vi "Report.vi"() -> ()   [LabVIEW 2020, in "Database Lib.lvlib"]
uses:
  Database Lib.lvlib
  <vilib>/Utility/miscctls.llb/LVRowAndColumnTypeDef.ctl
  <vilib>/Utility/NIReport.llb/Report Type.ctl
  <vilib>/addons/_office/_exclsub.llb/font.ctl
  <vilib>/addons/_office/excel.llb/Excel Easy Table (str).vi
  <vilib>/Utility/NIReport.llb/NI_report.lvclass
  <vilib>/Utility/NIReport.llb/NI_ReportGenerationCore.lvlib
  <vilib>/addons/_office/NI_ReportGenerationToolkit.lvlib
  <vilib>/Utility/NIReport.llb/Excel/NI_Excel.lvclass
panel:
  out "Grading Data":string[][](array[string])
  in  "Menu":enum32{"Log Catalog", "Log", "Grading"}(radio)
  out "Tab Control":enum32{"Log Catalog", "Log", "Grading"}(tab)
  in  "Search Log Catalog Table":bool
  out "Log Catalog Table":string[][](table)
  out "Log Table":string[][](table)
  in  "Save Log Table":bool
  in  "Search Log Table":bool
  in  "Catalog ID Log Table 2":u16 caption="Catalog ID" max=9999 step=1 format="%04.0f"
  in  "To Catalog ID Log Table":bool
  in  "Until Hour Log Table":u8 caption="Hour" max=23 step=1 format="%02.0f"
  in  "Until Minute Log Table":u8 caption="Minute" max=59 step=1 format="%02.0f"
  in  "Until Second Log Table":u8 caption="Second" max=59 step=1 format="%02.0f"
  in  "Until Time Log Table":bool
  in  "Since Time Log Table":bool
  in  "Until Date Log Table":bool
  in  "Until Year Log Table":u16 caption="Year" format="%04.0f"
  in  "Until Month Log Table":u8 caption="Month" max=12 step=1 format="%02.0f"
  in  "Until Day Log Table":u8 caption="Day" max=31 step=1 format="%02.0f"
  in  "Catalog ID Log Table 1":u16 caption="Catalog ID" max=9999 step=1 format="%04.0f"
  in  "Since Year Log Table":u16 caption="Year" format="%04.0f"
  in  "Since Month Log Table":u8 caption="Month" max=12 step=1 format="%02.0f"
  in  "Since Day Log Table":u8 caption="Day" max=31 step=1 format="%02.0f"
  in  "Since Hour Log Table":u8 caption="Hour" max=23 step=1 format="%02.0f"
  in  "Since Minute Log Table":u8 caption="Minute" max=59 step=1 format="%02.0f"
  in  "Since Second Log Table":u8 caption="Second" max=59 step=1 format="%02.0f"
  in  "Since Date Log Table":bool
  in  "From Catalog ID Log Table":bool
  out "Grading Table":string[][](table)
  in  "Search Grading Table":bool
  in  "Save Grading Table":bool
  in  "From Test Number":bool
  in  "Since Date Grading Table":bool
  in  "Since Second Grading Table":u8 caption="Second" max=59 step=1 format="%02.0f"
  in  "Since Minute Grading Table":u8 caption="Minute" max=59 step=1 format="%02.0f"
  in  "Since Hour Grading Table":u8 caption="Hour" max=23 step=1 format="%02.0f"
  in  "Since Day Grading Table":u8 caption="Day" max=31 step=1 format="%02.0f"
  in  "Since Month Grading Table":u8 caption="Month" max=12 step=1 format="%02.0f"
  in  "Since Year Grading Table":u16 caption="Year" format="%04.0f"
  in  "Test Number 1":u64 caption="Test Number" max=9999 step=1 format="%010.0f"
  in  "Until Day Grading Table":u8 caption="Day" max=31 step=1 format="%02.0f"
  in  "Until Month Grading Table":u8 caption="Month" max=12 step=1 format="%02.0f"
  in  "Until Year Grading Table":u16 caption="Year" format="%04.0f"
  in  "Until Date Grading Table":bool
  in  "Since Time Grading Table":bool
  in  "Until Time Grading Table":bool
  in  "Until Second Grading Table":u8 caption="Second" max=59 step=1 format="%02.0f"
  in  "Until Minute Grading Table":u8 caption="Minute" max=59 step=1 format="%02.0f"
  in  "Until Hour Grading Table":u8 caption="Hour" max=23 step=1 format="%02.0f"
  in  "To Test Number":bool
  in  "Test Number 2":u64 caption="Catalog ID" max=9999 step=1 format="%010.0f"
  in  "Graphs Grading Table":bool
  in  "Close":bool
  # "/"
  # "/"
  # ":"
  # ":"
  # "/"
  # "/"
  # ":"
  # ":"
  # "/"
  # "/"
  # ":"
  # ":"
  # "/"
  # "/"
  # ":"
  # ":"
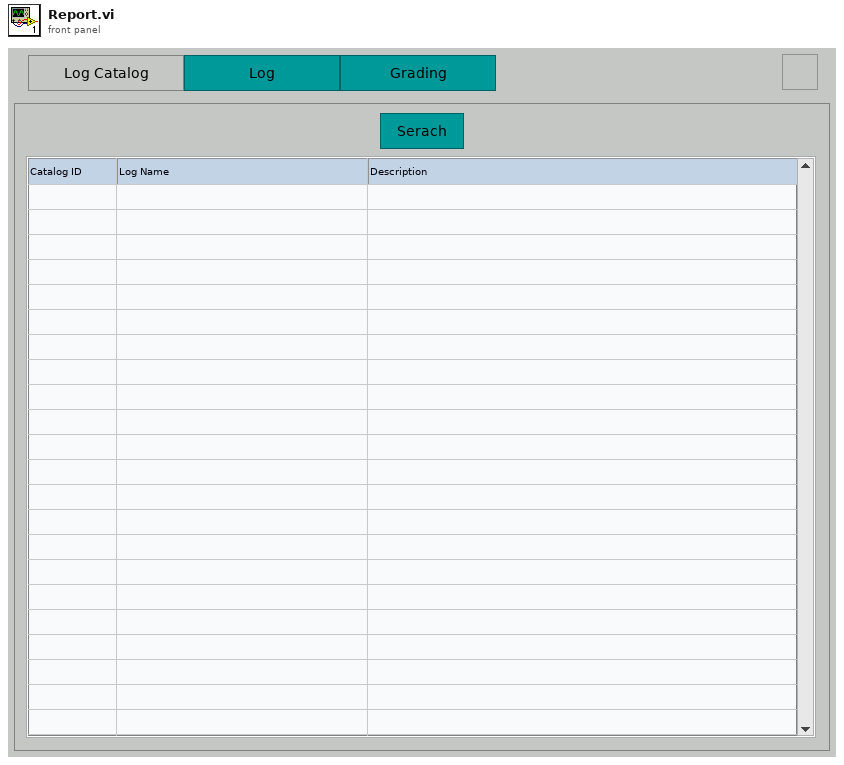
[diagram p1: front panel]
types:
  T1 = typedef "LVRowAndColumnTypeDef.ctl" = cluster{"Row":i32, "Column":i32}
  T2 = typedef "NI_ReportGenerationToolkit.lvlib/font.ctl" = cluster{"font name":string, "font size":dbl, "bold":u16, "italic":u16, "underline":u16, "strike through":u16, "font color":u32}
  T3 = enum16{"maximized", "minimized", "normal", "no change"}
  T4 = typedef "NI_ReportGenerationCore.lvlib/Report Type.ctl" = enum16{"HTML", "Word", "Excel"}
  T5 = cluster{"Since Year Grading Table":u16, "Since Month Grading Table":u8, "Since Day Grading Table":u8, "Until Year Grading Table":u16, "Until Month Grading Table":u8, "Until Day Grading Table":u8, "Since Date Grading Table":bool, "Until Date Grading Table":bool}
  T6 = cluster{"Since Hour Grading Table":u8, "Since Minute Grading Table":u8, "Since Second Grading Table":u8, "Until Hour Grading Table":u8, "Until Minute Grading Table":u8, "Until Second Grading Table":u8, "Since Time Grading Table":bool, "Until Time Grading Table":bool}
  T7 = cluster{"Test Number 1":u64, "Test Number 2":u64, "From Test Number":bool, "To Test Number":bool}
  T8 = cluster{"Since Year Log Table":u16, "Since Month Log Table":u8, "Since Day Log Table":u8, "Until Year Log Table":u16, "Until Month Log Table":u8, "Until Day Log Table":u8, "Since Date Log Table":bool, "Until Date Log Table":bool}
  T9 = cluster{"Since Hour Log Table":u8, "Since Minute Log Table":u8, "Since Second Log Table":u8, "Until Hour Log Table":u8, "Until Minute Log Table":u8, "Until Second Log Table":u8, "Since Time Log Table":bool, "Until Time Log Table":bool}
  T10 = cluster{"Catalog ID Log Table 1":u16, "Catalog ID Log Table 2":u16, "From Catalog ID Log Table":bool, "To Catalog ID Log Table":bool}
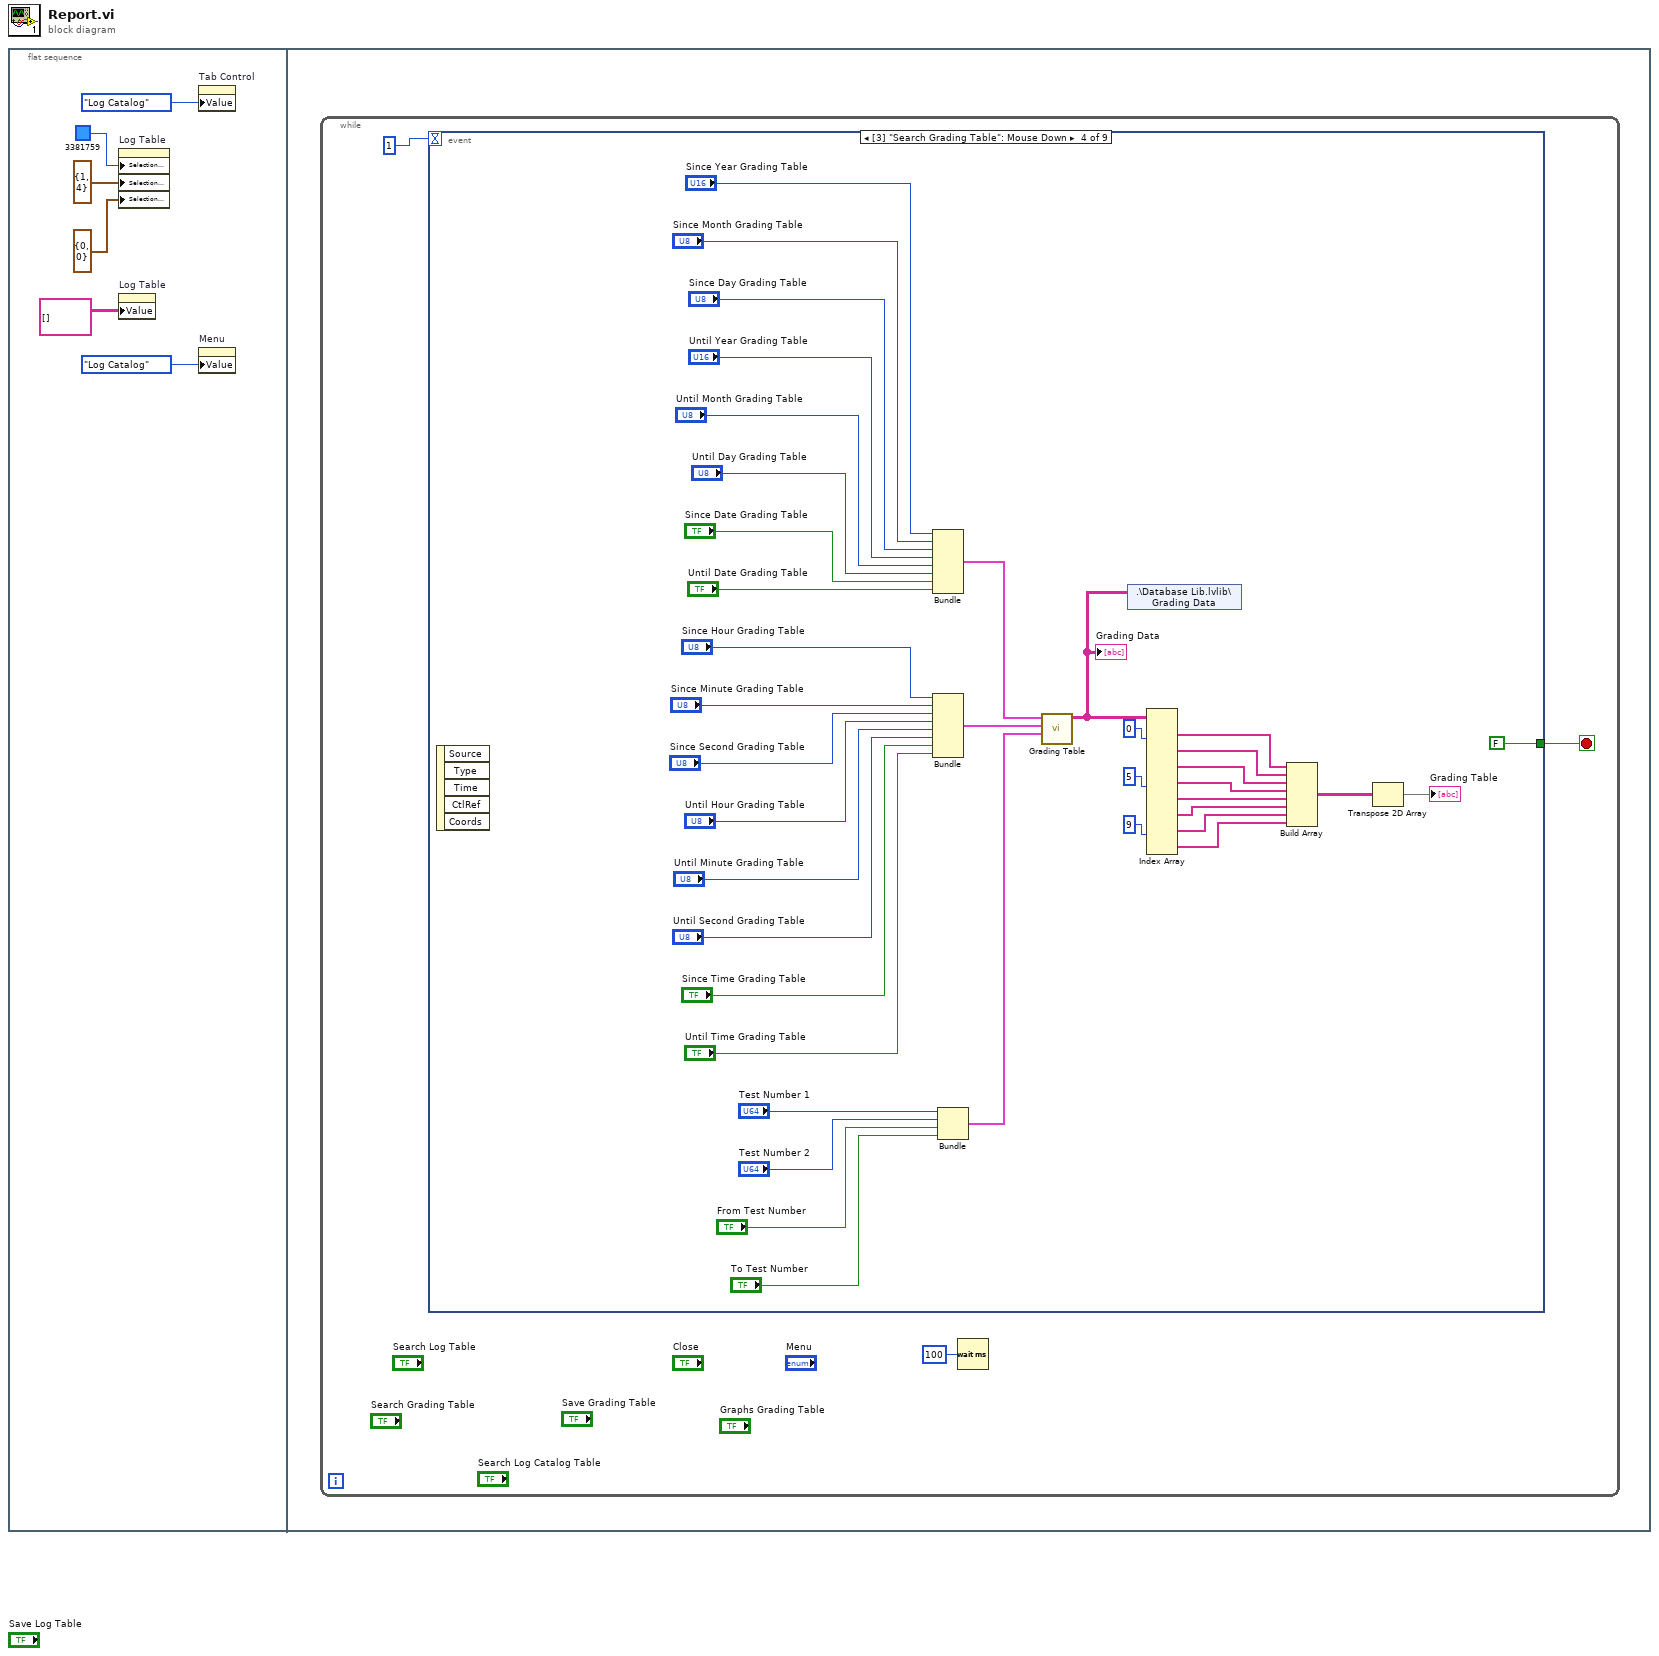
[diagram p0: block diagram]
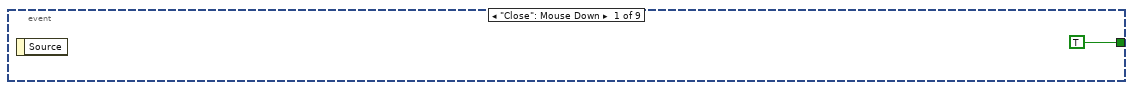
[diagram p2: hidden frame]
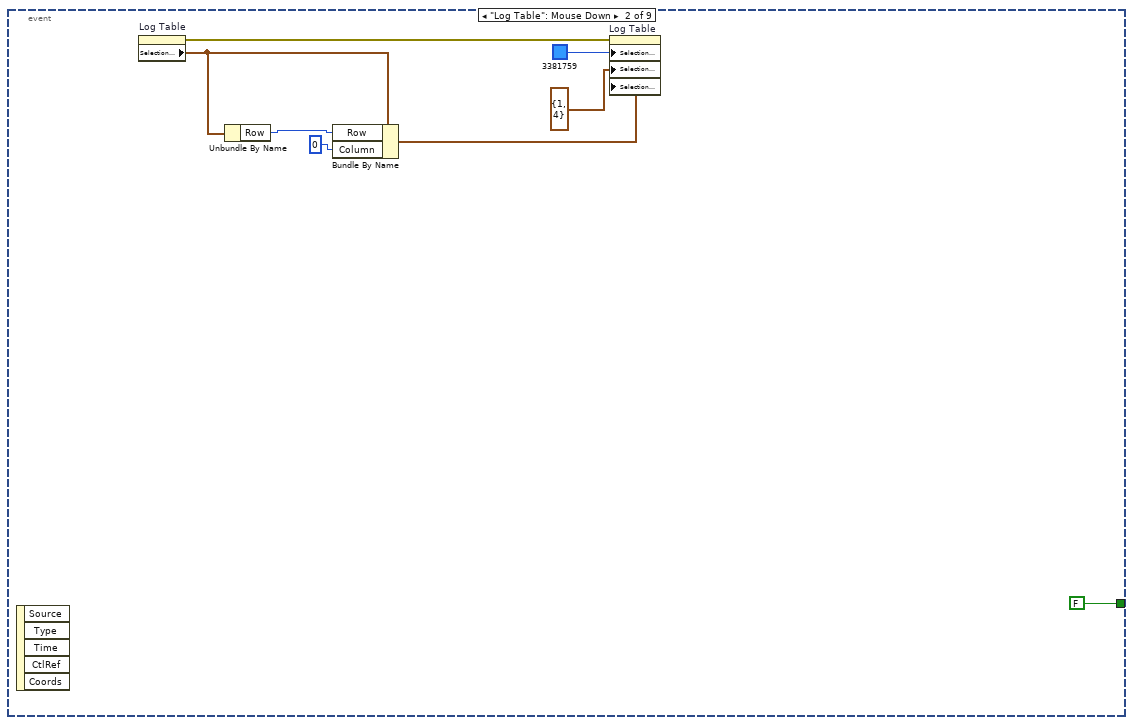
[diagram p3: hidden frame]
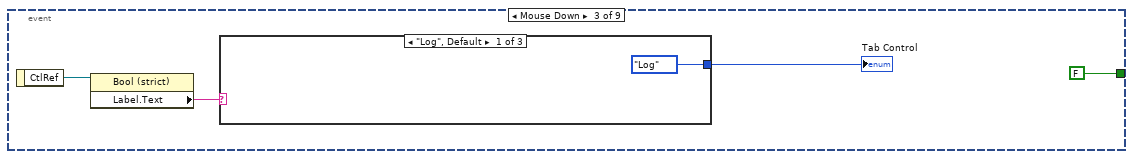
[diagram p4: hidden frame]
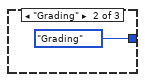
[diagram p5: hidden frame]
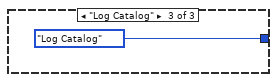
[diagram p6: hidden frame]
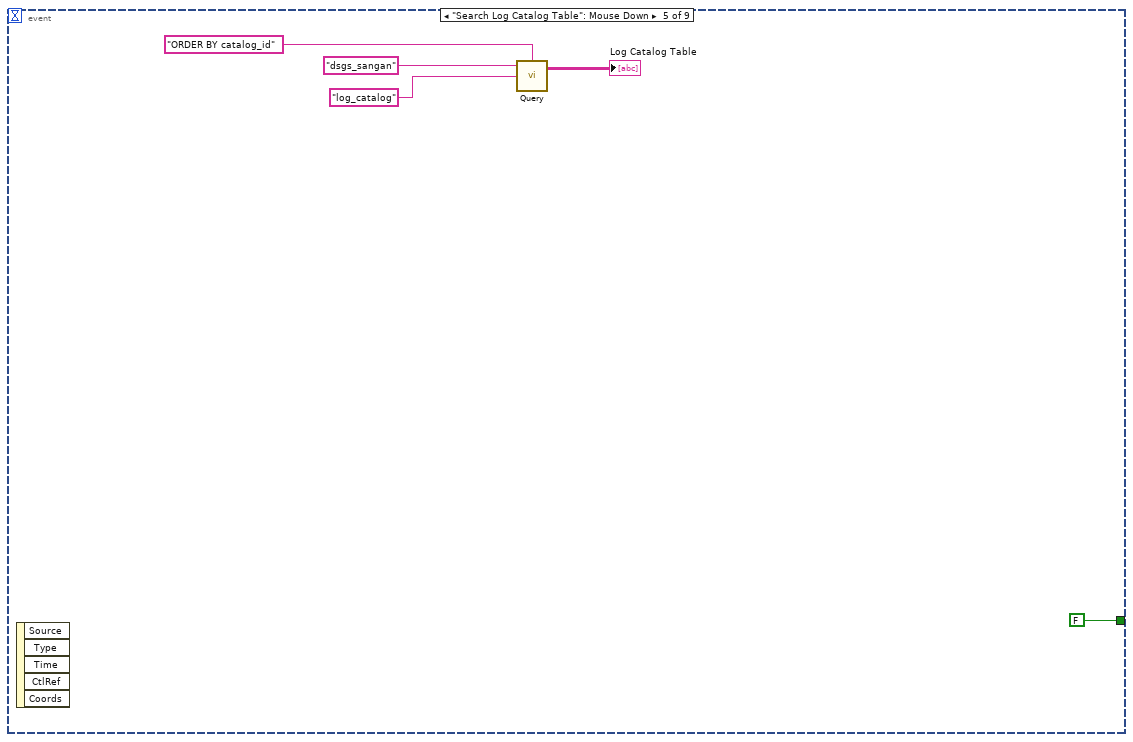
[diagram p7: hidden frame]
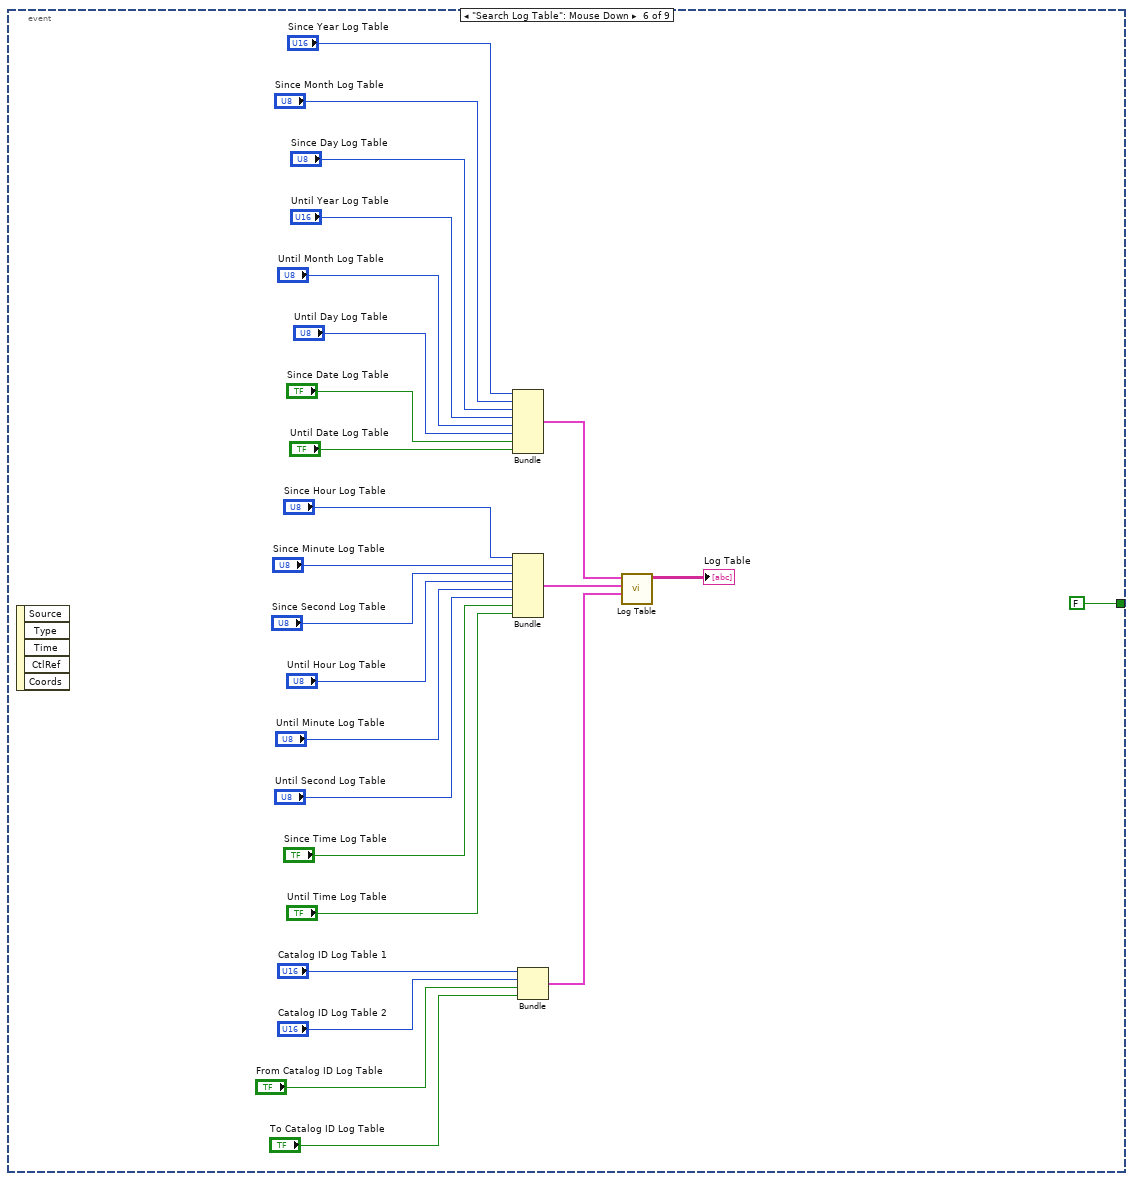
[diagram p8: hidden frame]
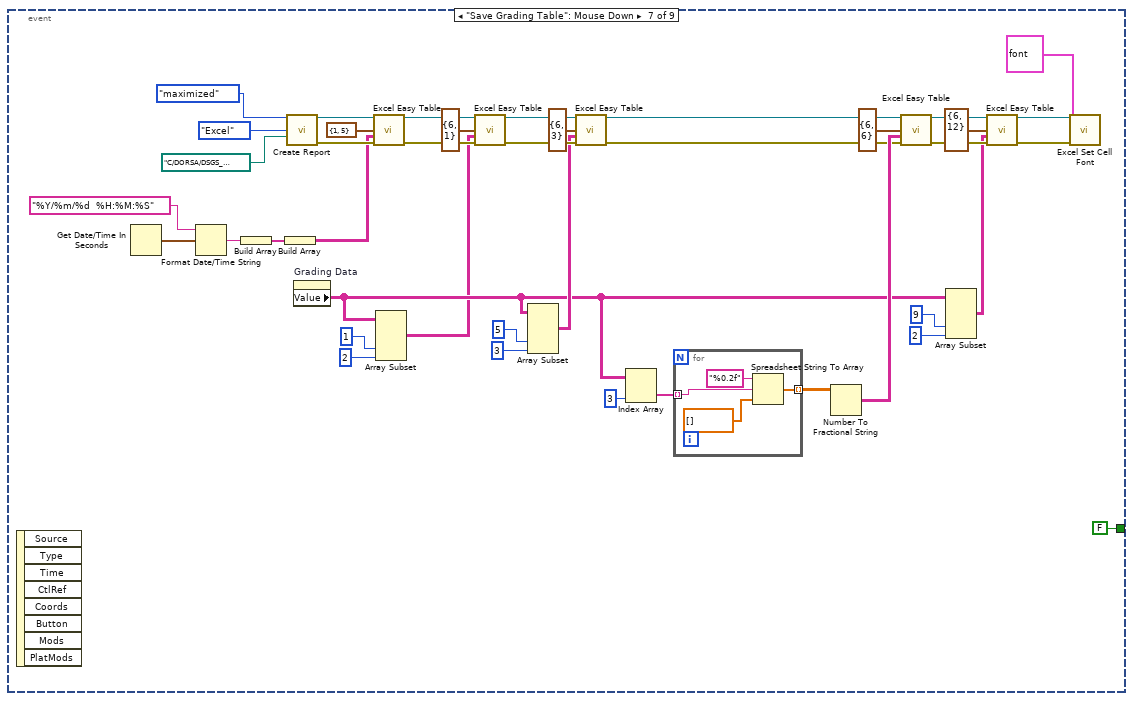
[diagram p9: hidden frame]
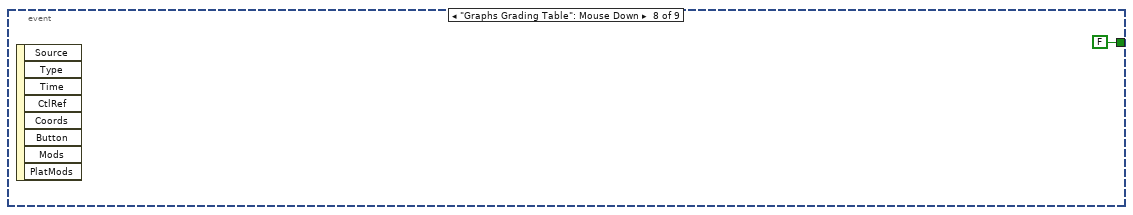
[diagram p10: hidden frame]
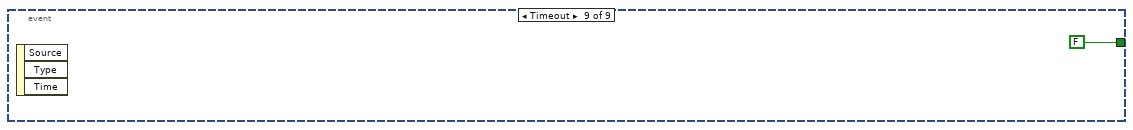
[diagram p11: hidden frame]
diagram:
  n1 = flat-sequence {
    frame #0 {
      n2 = property on="Log Table" class="Tbl (strict)"("Selection Color"=u32 3381759, "Selection Size"=T1 {"Row"=1, "Column"=4}, "Selection Start"=T1 {"Row"=0, "Column"=0}) -> ()  [unwired: 2 in, 2 out]
      n3 = property on="Log Table" class="Tbl (strict)"("Value"=string[][] []) -> ()  [unwired: 2 in, 2 out]
      n4 = property on="Tab Control" class="TabCtl (strict)"("Value"=enum32{"Log Catalog", "Log", "Grading"}."Log Catalog" ("Tab Control")) -> ()  [unwired: 2 in, 2 out]
      n5 = property on="Menu" class="RadioBtnsControl (strict)"("Value"=enum32{"Log Catalog", "Log", "Grading"}."Log Catalog" ("Menu")) -> ()  [unwired: 2 in, 2 out]
    }
    frame #1 {
      n6 = while {
        stop <- w9 stop-if-true
        n7 = event shown="[3] \"Search Grading Table\": Mouse Down" {
          selector: _ -> [_ _ _ _ _ _ _ _ _]
          dyn-events: _ -> [_ _ _ _ _ _ _ _ _]
          timeout: 1 -> [_ _ _ _ _ _ _ _ _]
          tunnel: [TRUE FALSE FALSE FALSE FALSE FALSE FALSE FALSE FALSE] -> w9
          event "Close": Mouse Down {
            n8 = event-data() -> ()  [unwired: 1 in, 1 out]
          }
          event "Log Table": Mouse Down {
            n9 = event-data() -> ()  [unwired: 1 in, 5 out]
            n10 = property on="Log Table" class="Tbl (strict)"() -> (error out=w16:errorcluster, "Selection Start"=w14:T1)  [unwired: 2 in, 1 out]
            n11 = Unbundle By Name(w14) -> ("Row"=w15:i32)
            n12 = Bundle By Name(cluster=w14, "Row"=w15, "Column"=0) -> (w17:T1)
            n13 = property on="Log Table" class="Tbl (strict)"(error in=w16, "Selection Color"=u32 3381759, "Selection Size"=T1 {"Row"=1, "Column"=4}, "Selection Start"=w17) -> ()  [unwired: 1 in, 2 out]
          }
          event "Menu.Log Catalog", "Menu.Log", "Menu.Grading": Mouse Down {
            n14 = event-data() -> ("CtlRef"=w21:refnum<vi>)  [unwired: 1 in]
            n15 = property class="Bool (strict)"(reference=w21) -> ("Label.Text"=w20:string)  [unwired: 1 in, 2 out]
            n16 = case shown="\"Log\", Default" w20 {
              tunnel: [enum32{"Log Catalog", "Log", "Grading"}."Log" ("Tab Control") enum32{"Log Catalog", "Log", "Grading"}."Grading" ("Tab Control") enum32{"Log Catalog", "Log", "Grading"}."Log Catalog" ("Tab Control")] -> w19
              frame "Log", Default {
              }
              frame "Grading" {
              }
              frame "Log Catalog" {
              }
            }
            "Tab Control" <- w19
          }
          event "Search Grading Table": Mouse Down {
            n17 = event-data() -> ()  [unwired: 1 in, 5 out]
            n18 = Bundle("Since Year Grading Table"="Since Year Grading Table", "Since Month Grading Table"="Since Month Grading Table", "Since Day Grading Table"="Since Day Grading Table", "Until Year Grading Table"="Until Year Grading Table", "Until Month Grading Table"="Until Month Grading Table", "Until Day Grading Table"="Until Day Grading Table", "Since Date Grading Table"="Since Date Grading Table", "Until Date Grading Table"="Until Date Grading Table") -> (w61:T5)  [unwired: 1 in]
            n19 = Bundle("Since Hour Grading Table"="Since Hour Grading Table", "Since Minute Grading Table"="Since Minute Grading Table", "Since Second Grading Table"="Since Second Grading Table", "Until Hour Grading Table"="Until Hour Grading Table", "Until Minute Grading Table"="Until Minute Grading Table", "Until Second Grading Table"="Until Second Grading Table", "Since Time Grading Table"="Since Time Grading Table", "Until Time Grading Table"="Until Time Grading Table") -> (w62:T6)  [unwired: 1 in]
            n20 = Bundle("Test Number 1"="Test Number 1", "Test Number 2"="Test Number 2", "From Test Number"="From Test Number", "To Test Number"="To Test Number") -> (w63:T7)  [unwired: 1 in]
            n21 = call "Grading Table.vi"("Test number"=w63, "Time"=w62, "Date"=w61) -> ("Grading Table"=w26:string[][])  [unwired: 7 in, 1 out]
            "Grading Data" <- w26
            n22 = shared-variable ".\\Database Lib.lvlib\\Grading Data"(w26) -> ()  [unwired: 1 in, 1 out]
            n23 = Index Array(array=w26, index (col) #1=0 ("disabled index (col)"), index (col) #4=5 ("index (col)"), index (col) #7=9 ("index (col)")) -> (element #1=w37:string[], element #2=w36:string[], element #3=w35:string[], element #4=w34:string[], element #5=w33:string[], element #6=w32:string[], element #7=w31:string[], element #8=w30:string[])  [unwired: 13 in]
            n24 = Build Array(w37, w36, w35, w34, w33, w32, w31, w30) -> (w29:string[][])
            n25 = Transpose 2D Array(2D array=w29) -> (transposed array=→"Grading Table":string[][])
          }
          event "Search Log Catalog Table": Mouse Down {
            n26 = event-data() -> ()  [unwired: 1 in, 5 out]
            n27 = call "Query.vi"("Condition"="ORDER BY catalog_id", "Table Name"="log_catalog", "Connection Name"="dsgs_sangan") -> ("data"=→"Log Catalog Table":string[][])  [unwired: 1 in, 1 out]
          }
          event "Search Log Table": Mouse Down {
            n28 = event-data() -> ()  [unwired: 1 in, 5 out]
            n29 = Bundle("Since Year Log Table"="Since Year Log Table", "Since Month Log Table"="Since Month Log Table", "Since Day Log Table"="Since Day Log Table", "Until Year Log Table"="Until Year Log Table", "Until Month Log Table"="Until Month Log Table", "Until Day Log Table"="Until Day Log Table", "Since Date Log Table"="Since Date Log Table", "Until Date Log Table"="Until Date Log Table") -> (w76:T8)  [unwired: 1 in]
            n30 = Bundle("Since Hour Log Table"="Since Hour Log Table", "Since Minute Log Table"="Since Minute Log Table", "Since Second Log Table"="Since Second Log Table", "Until Hour Log Table"="Until Hour Log Table", "Until Minute Log Table"="Until Minute Log Table", "Until Second Log Table"="Until Second Log Table", "Since Time Log Table"="Since Time Log Table", "Until Time Log Table"="Until Time Log Table") -> (w75:T9)  [unwired: 1 in]
            n31 = Bundle("Catalog ID Log Table 1"="Catalog ID Log Table 1", "Catalog ID Log Table 2"="Catalog ID Log Table 2", "From Catalog ID Log Table"="From Catalog ID Log Table", "To Catalog ID Log Table"="To Catalog ID Log Table") -> (w70:T10)  [unwired: 1 in]
            n32 = call "Log Table.vi"("Catalog ID"=w70, "Time"=w75, "Date"=w76) -> ("Log Table"=→"Log Table":string[][])  [unwired: 7 in, 1 out]
          }
          event "Save Grading Table": Mouse Down {
            n33 = event-data() -> ()  [unwired: 1 in, 8 out]
            n34 = Get Date/Time In Seconds() -> (seconds since 1Jan1904=w123:timestamp)
            n35 = Format Date/Time String(time format string (%c)="%Y/%m/%d  %H:%M:%S", seconds (now)=w123) -> (date/time string=w121:string)  [unwired: 1 in]
            n36 = Build Array(w121) -> (w120:string[])
            n37 = Build Array(w120) -> (w119:string[][])
            n38 = call <vilib>:"Create Report.vi"("window state (normal)"=T3."maximized", "report type"=Report_Type."Excel", "template (empty)"=path "C:/DORSA/DSGS_Sangan/Grading Report Template.xltx") -> ("report out"=w127:refnum<class "NI_report.lvclass">, "error out"=w131:errorcluster)  [unwired: 11 in]
            n39 = property on="Grading Data" class="Arr (strict)"() -> ("Value"=w96:string[][])  [unwired: 2 in, 2 out]
            n40 = call-poly <vilib>:"Excel Easy Table.vi"("report in"=w127, "start (0, 0)"=cluster{"row":i32, "column":i32} {"row"=1, "column"=5}, "text data"=w119, "error in (no error)"=w131) -> ("report out"=w126:refnum<class "NI_report.lvclass">, "error out"=w130:errorcluster)  [unwired: 7 in, 3 out]
            n41 = Array Subset(array=w96, index (col)=1 ("index"), length (col)=2 ("length")) -> (w94:string[][])  [unwired: 2 in]
            n42 = call-poly <vilib>:"Excel Easy Table.vi"("report in"=w126, "start (0, 0)"=cluster{"row":i32, "column":i32} {"row"=6, "column"=1}, "text data"=w94, "error in (no error)"=w130) -> ("report out"=w125:refnum<class "NI_report.lvclass">, "error out"=w129:errorcluster)  [unwired: 7 in, 3 out]
            n43 = Array Subset(array=w96, index (col)=5 ("index"), length (col)=3 ("length")) -> (w113:string[][])  [unwired: 2 in]
            n44 = call-poly <vilib>:"Excel Easy Table.vi"("report in"=w125, "start (0, 0)"=cluster{"row":i32, "column":i32} {"row"=6, "column"=3}, "text data"=w113, "error in (no error)"=w129) -> ("report out"=w107:refnum<class "NI_report.lvclass">, "error out"=w105:errorcluster)  [unwired: 7 in, 3 out]
            n45 = Index Array(array=w96, index (col)=3 ("disabled index (col)")) -> (element=w109:string[])  [unwired: 1 in]
            n46 = for {
              tunnel: w109 -> [w138] mode=indexing
              tunnel: [w135] -> w108 mode=indexing
              n47 = Spreadsheet String To Array(format string="%0.2f", spreadsheet string=w138, array type (2D Dbl)=dbl[] []) -> (array=w135:dbl[])  [unwired: 1 in]
            }
            n48 = Number To Fractional String(number=w108) -> (F-format string=w106:string[][])  [unwired: 3 in]
            n49 = call-poly <vilib>:"Excel Easy Table.vi"("report in"=w107, "start (0, 0)"=cluster{"row":i32, "column":i32} {"row"=6, "column"=6}, "text data"=w106, "error in (no error)"=w105) -> ("report out"=w103:refnum<class "NI_report.lvclass">, "error out"=w100:errorcluster)  [unwired: 7 in, 3 out]
            n50 = Array Subset(array=w96, index (col)=9 ("index"), length (col)=2 ("length")) -> (w95:string[][])  [unwired: 2 in]
            n51 = call-poly <vilib>:"Excel Easy Table.vi"("report in"=w103, "start (0, 0)"=cluster{"row":i32, "column":i32} {"row"=6, "column"=12}, "text data"=w95, "error in (no error)"=w100) -> ("report out"=w102:refnum<class "NI_report.lvclass">, "error out"=w101:errorcluster)  [unwired: 7 in, 3 out]
            n52 = call <vilib>:"Excel Set Cell Font.vi"("report in"=w102, "font"=T2 {"font name"="Times New Roman", "font size"=11.0, "bold"=0, "italic"=0, "underline"=0, "strike through"=0, "font color"=16777216}, "error in (no error)"=w101) -> ()  [unwired: 11 in, 2 out]
          }
          event "Graphs Grading Table": Mouse Down {
            n53 = event-data() -> ()  [unwired: 1 in, 8 out]
          }
          event Timeout {
            n54 = event-data() -> ()  [unwired: 1 in, 3 out]
          }
        }
        n55 = Wait (ms)(milliseconds to wait=u32 100) -> ()  [unwired: 1 out]
      }
    }
  }
